vi "CreateNewBoard.vi"(8 "error in (no error)":errorcluster, 10 "Size":T1) -> (0 "error out":errorcluster, 3 "Board out":refnum<class "Board.lvclass">)   [LabVIEW 2015, in "TronviewGame.lvlib" / "Board.lvclass"]
uses:
  Board.lvclass
  BoardSize.ctl
  FieldState.ctl
  Board.lvclass/Board.ctl
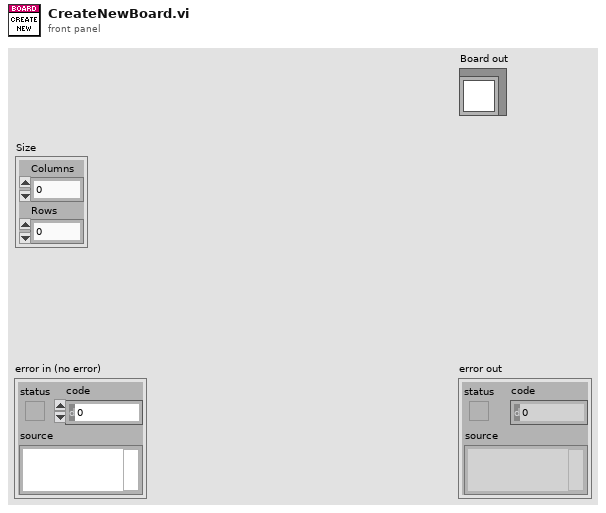
[diagram p1: front panel]
types:
  T1 = typedef "TronviewGame.lvlib/Board.lvclass/BoardSize.ctl" = cluster{"Columns":u16, "Rows":u16}
  T2 = typedef "TronviewGame.lvlib/Board.lvclass/FieldState.ctl" = enum16{"Empty", "Blocked", "Player1Position", "Player2Postion", "Player1Marked", "Player2Marked"}
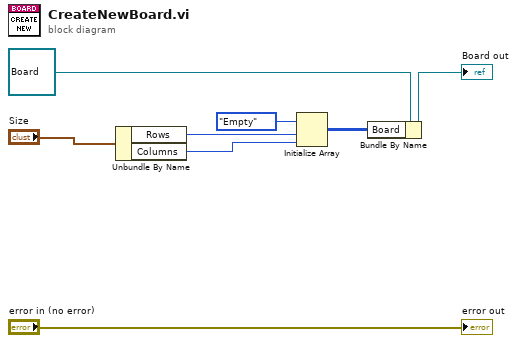
[diagram p0: block diagram]
diagram:
  n1 = Unbundle By Name("Size") -> ("Rows"=w4:u16, "Columns"=w3:u16)
  n2 = Initialize Array(FieldState."Empty" ("FieldState"), w4, w3) -> (w6:T2[][])
  n3 = Bundle By Name(cluster=refnum<class "Board.lvclass"> refnum ("Board in"), "Board"=w6) -> (→"Board out":refnum<class "Board.lvclass">)
  "error out" <- "error in (no error)"
